vi "Simple_DAQ_AnalogIO.get channel voltage.vi"(0 "i ref in":refnum<vi>, 3 "Timeout":i32=10000, 5 "error in":errorcluster caption="Fehler (Eingang, kein Fehler)", 9 "channel_index":i32) -> (11 "voltage":dbl, 14 "i ref out":refnum<vi>, 17 "timed out":bool, 19 "error out":errorcluster caption="Fehler (Ausgang)")   [LabVIEW 2014, in "Simple_DAQ_AnalogIO.lvlib"]
doc: "Contact: Falk Ziegler, eMail: info@lab-coding.de"
uses:
  Simple_DAQ_AnalogIO.lvlib
  CS_Core/CSSystem/CoreDefs/CoreDefs.error_type.ctl
  CS_Core/CSApplicationBaseClasses/PSChannelBase/PSChannelBase.directionType.ctl
  CS_Core/CSApplicationBaseClasses/PSChannelBase/PSChannelBase.serviceType.ctl
  CSlibraries/UtilityLib/UtilityLib.valueStatus.ctl
  <vilib>/DAQmx/read.llb/DAQmx Read (Analog DBL 1Chan 1Samp).vi
  CS_Core/CSSystem/CoreLib/CoreLib.lvlib
  CSlibraries/UtilityLib/UtilityLib.lvlib
  CS_Core/CSApplicationBaseClasses/DeviceBase/DeviceBase.lvlib
  CS_Core/CSApplicationBaseClasses/PSChannelBase/PSChannelBase.lvlib
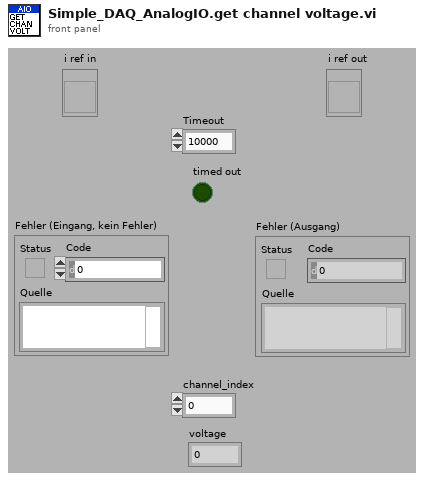
[diagram p1: front panel]
types:
  T1 = typedef "CoreDefs.error_type.ctl" = enum16{"no error", "can't load process", "can't unload process", "process does not exist", "can't install process", "can't remove process", "unknown function", "time out", "can't execute function", "duplicate queue name", "super not found", "caller queue invalid", "can't ping process", "unknown error", "VISA Error", "VISA timeout", "GPIB timeout", "GPIB error", "communication error", "data type mismatch", "can't read data from OPC server", "can't write data to OPC server", "OET error", "function not implemented", "process already exists", "invalid Shared Variable name", "error writing Shared Variable", "error reading Shared Variable", "invalid client name", "corrupt database", "unknown class", "call not authorized", "parameter out of range", "OET timeout: can't get data to modify", "invalid queue name", "requested operation incompatible with current state", "event undefined", "event disabled", "state undefined", "caller is not a friend", "EventBuilder: bad eventID", "EventBuilder: no DAQ devices", "a thread must not stop itself", "UNUSED ELEMENT4", "DiscArchiver: eventData incomplete", "DiscArchiver: eventData does not belong to run", "DiscArchiver: can't open file", "DiscArchiver: can't write to file", "DiscArchiver: available disc space low", "can't acquire semaphore", "error reading data from database", "notifier object is not existing", "can't register process", "can't unregister process", "illegal event type", "object disabled", "object already exists", "can't change state", "Instrument not found", "no connection to remote node", "invalid reference", "N/A", "UNUSED ELEMENT 1", "element not found", "illegal TCP/IP connection detected", "object does not exist", "invalid access ID", "unknown CS system", "invalid privilige", "unsupported data type", "unsupported server type", "IO server already exists", "Shared Variable already exists"}
  T2 = typedef "PSChannelBase.lvlib/PSChannelBase.serviceType.ctl" = enum16{"onOff", "voltage", "current", "tripCurrent", "rampUpSpeed", "rampDownSpeed", "status"}
  T3 = typedef "PSChannelBase.lvlib/PSChannelBase.directionType.ctl" = enum16{"unknown", "update actual value", "update nominal value", "update both"}
  T4 = typedef "UtilityLib.lvlib/UtilityLib.valueStatus.ctl" = enum16{"no info available", "stand by/off", "on", "warning", "alarm/malfunction", "not implemented", "user action required", "important information", "system default", "control default", "indicator default", "button default"}
  T5 = typedef "Simple_DAQ_AnalogIO.lvlib/Simple_DAQ_AnalogIO.i attribute.ctl" = cluster{"inputs":cluster{"index":i32[], "channel_task":refnum<k21>[], "range":cluster{"min":dbl, "max":dbl}[], "channel_number":i32, "scale_factor":dbl}, "outputs":cluster{"index":i32[], "channel_task":refnum<k21>[], "range":cluster{"min":dbl, "max":dbl}[], "channel_number":i32, "scale_factor":dbl}}
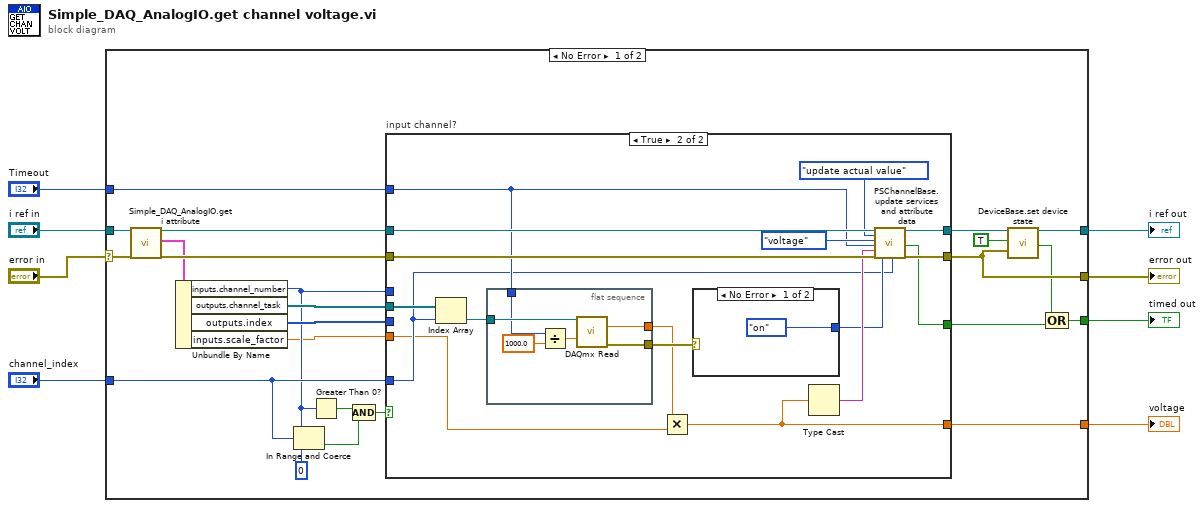
[diagram p0: block diagram]
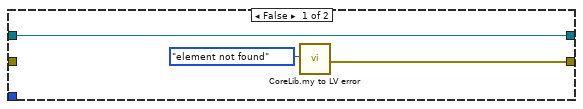
[diagram p2: hidden frame]
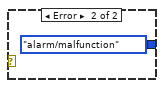
[diagram p3: hidden frame]
diagram:
  n1 = case shown="No Error" "error in" {
    selector: "error in" -> [w30 w60]
    tunnel: "i ref in" -> [w31 w61]
    tunnel: [w22 w61] -> w6
    tunnel: "Timeout" -> [w24 _]
    tunnel: "channel_index" -> [w15 _]
    tunnel: [w16 _] -> w3
    tunnel: [w20 _] -> w2
    tunnel: [w19 w60] -> w1
    frame No Error {
      n2 = call "Simple_DAQ_AnalogIO.get i attribute.vi"("i ref in"=w31, "error in (no error)"=w30) -> ("i ref out"=w29:refnum<vi>, "i attribute"=w27:T5, "error out"=w28:errorcluster)  [unwired: 15 in]
      n3 = Unbundle By Name(w27) -> ("inputs.channel_number"=w10:i32, "outputs.channel_task"=w26:refnum<k21>[], "outputs.index"=w25:i32[], "inputs.scale_factor"=w9:dbl)
      n4 = In Range and Coerce(upper limit=w10, x=w15, lower limit=0) -> (In Range?=w13:bool)  [unwired: 1 out]
      n5 = Greater Than 0?(x=w10) -> (x > 0?=w11:bool)
      n6 = Compound Arithmetic op=AND(w11, w13) -> (w12:bool)
      n7 = case "input channel?" shown="True" w12 {
        tunnel: w29 -> [w33 w50]
        tunnel: w28 -> [_ w47]
        tunnel: w26 -> [_ w51]
        tunnel: w25 -> [_ _]
        tunnel: w24 -> [_ w39]
        tunnel: [w33 w49] -> w23
        tunnel: [w34 w48] -> w19
        tunnel: [_ w46] -> w17
        tunnel: [_ w35] -> w20
        tunnel: w15 -> [_ w38]
        tunnel: w10 -> [_ _]
        tunnel: w9 -> [_ w36]
        frame False {
          n8 = call "CoreLib.my to LV error.vi"("ErrorTypes"=CoreDefs.error_type."element not found") -> ("myErrorCluster"=w34:errorcluster)  [unwired: 17 in, 1 out]
        }
        frame True {
          n9 = Index Array(array=w51, index=w38) -> (element=w45:refnum<k21>)
          n10 = flat-sequence {
            tunnel: w45 -> [w59]
            tunnel: [w58] -> w43
            tunnel: [w57] -> w37
            tunnel: w39 -> [w55]
            frame #0 {
              n11 = Divide(x=w55, y=1000.0) -> (x/y=w56:dbl)
              n12 = call-poly <vilib>:"DAQmx Read.vi"("task/channels in"=w59, "timeout"=w56) -> ("data"=w57:dbl, "error out"=w58:errorcluster)  [unwired: 11 in, 1 out]
            }
          }
          n13 = Multiply(x=w37, y=w36) -> (x*y=w35:dbl)
          n14 = case shown="No Error" w43 {
            tunnel: [UtilityLib.valueStatus."on" ("quality") UtilityLib.valueStatus."alarm/malfunction" ("quality")] -> w42
            frame No Error {
            }
            frame Error {
            }
          }
          n15 = Type Cast(x=w35) -> (*(type *) &x=w44:string)  [unwired: 1 in]
          n16 = call "PSChannelBase.update services and attribute data.vi"("i ref in"=w50, "direction"=PSChannelBase.directionType."update actual value", "service"=PSChannelBase.serviceType."voltage", "ms timeout (10000)"=w39, "value"=w44, "error in (no error)"=w47, "quality"=w42, "channelNumber"=w38) -> ("i ref out"=w49:refnum<vi>, "timed out"=w46:bool, "error out"=w48:errorcluster)  [unwired: 9 in]
        }
      }
      n17 = call "DeviceBase.set device state.vi"("i ref in"=w23, "implicit"=TRUE, "device error"=w19) -> ("i ref out"=w22:refnum<vi>, "timed out"=w18:bool)  [unwired: 14 in, 1 out]
      n18 = Compound Arithmetic op=OR(w18, w17) -> (w16:bool)
    }
    frame Error {
    }
  }
  "error out" <- w1
  "timed out" <- w3
  "i ref out" <- w6
  "voltage" <- w2
